vi "Initialize System (Single Bus Multiple Lines).vi"(0 "bus configuration":T1={"nominal voltage [V]"=230.0, "nominal frequency"=enum."50 Hz", "samples per cycle"=192, "type of reference voltage"=enum."Constant", "symmetrical components calculation"=1, "voltage channels"=[], "current channels"=[]} {"current channels"."physical channels"."channel phase" items=["Phase A (L1)", "Phase B (L2)", "Phase C (L3)", "Phase N (Neutral)"]; "voltage channels"."physical channels"."channel phase" items=["Phase A (L1)", "Phase B (L2)", "Phase C (L3)", "Phase N (Neutral)"]; "symmetrical components calculation" items=["Phase to Phase", "Phase to Neutral"]; "samples per cycle" min=128 max=512}, 11 "error in (no error)":errorcluster) -> (4 "nominal sample rate [Hz]":u16, 10 "system info out":refnum<class "EP System Info.lvclass">, 15 "error out":errorcluster)   [LabVIEW 2014, in "NI_EP_Power Quality.lvlib"]
doc: "Sets the basic configuration of the electrical power system based on different line and bus configurations. You must manually select the polymorphic instance you want to use."
uses:
  <vilib>/addons/Electrical Power/PQ/NI_EP_Power Quality.lvlib
  <vilib>/addons/Electrical Power/PQ/Common/Classes/System Info/EP System Info.lvclass
  <vilib>/addons/Electrical Power/PQ/Common/Controls/ep_Bus Config.ctl
  <vilib>/addons/Electrical Power/PQ/Common/Controls/ep_Symmetrical Component Calculation.ctl
  <vilib>/addons/Electrical Power/PQ/Common/Controls/ep_Channels Config.ctl
  <vilib>/addons/Electrical Power/PQ/Common/Controls/ep_Channel Phase.ctl
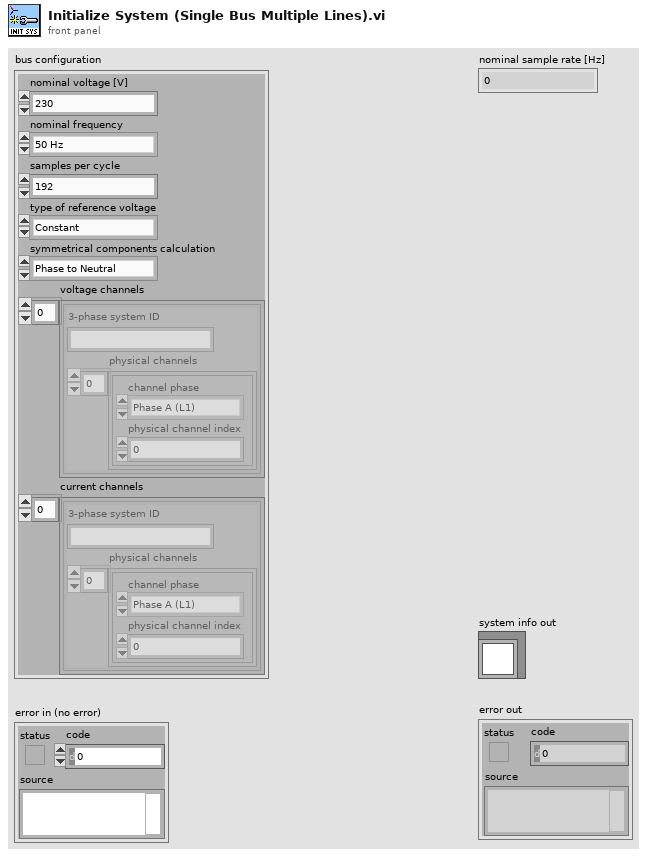
[diagram p1: front panel]
types:
  T1 = typedef "NI_EP_Power Quality.lvlib/ep_Bus Config.ctl" = cluster{"nominal voltage [V]":dbl, "nominal frequency":enum16{"50 Hz", "60 Hz"}, "samples per cycle":u16, "type of reference voltage":enum16{"Constant", "Sliding"}, "symmetrical components calculation":T2, "voltage channels":T3[], "current channels":T3[]}
  T2 = typedef "NI_EP_Power Quality.lvlib/ep_Symmetrical Component Calculation.ctl" = u16
  T3 = typedef "NI_EP_Power Quality.lvlib/ep_Channels Config.ctl" = cluster{"3-phase system ID":string, "physical channels":cluster{"channel phase":T4, "physical channel index":u16}[]}
  T4 = typedef "NI_EP_Power Quality.lvlib/ep_Channel Phase.ctl" = u16
  T5 = typedef "NI_EP_Power Quality.lvlib/ep_Channel Ranges.ctl" = cluster{"3-phase system ID":string, "ranges":dbl[]}
  T6 = typedef "NI_EP_Power Quality.lvlib/ep_Channel Sensitivity.ctl" = cluster{"3-phase system ID":string, "sensitivity":dbl[]}
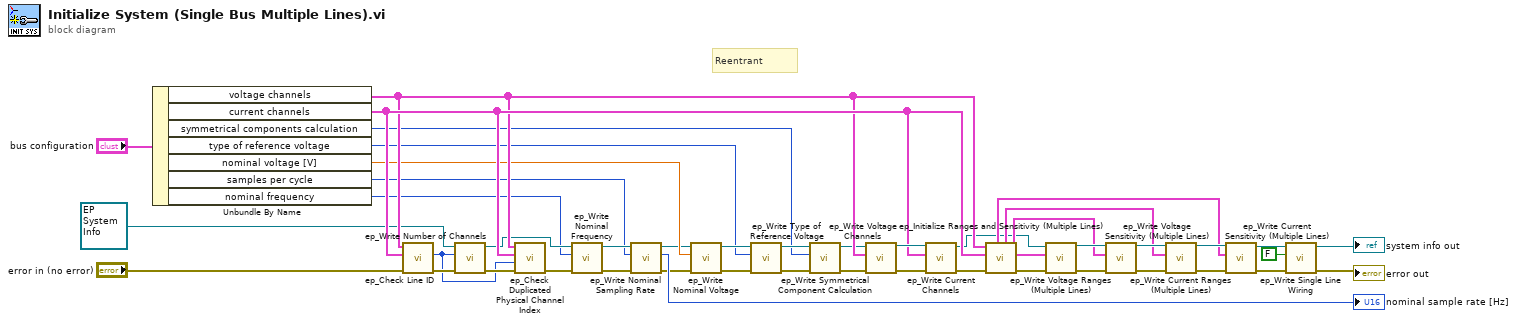
[diagram p0: block diagram]
diagram:
  # "Reentrant"
  n1 = Unbundle By Name("bus configuration") -> ("voltage channels"=w34:T3[], "current channels"=w35:T3[], "symmetrical components calculation"=w10:T2, "type of reference voltage"=w21:enum16{"Constant", "Sliding"}, "nominal voltage [V]"=w22:dbl, "samples per cycle"=w2:u16, "nominal frequency"=w7:enum16{"50 Hz", "60 Hz"})
  n2 = call <vilib>:"ep_Check Line ID.vi"("error in (no error)"="error in (no error)", "current channels"=w35, "voltage channels"=w34) -> ("error out"=w18:errorcluster, "number of channels"=w15:i32)  [unwired: 7 in]
  n3 = call <vilib>:"ep_Write Number of Channels.vi"("error in (no error)"=w18, "number of channels"=w15, "system info in"=refnum<class "EP System Info.lvclass"> refnum ("EP System Info.lvclass")) -> ("error out"=w17:errorcluster, "system info out"=w8:refnum<class "EP System Info.lvclass">)  [unwired: 7 in]
  n4 = call <vilib>:"ep_Check Duplicated Physical Channel Index.vi"("error in (no error)"=w17, "number of channels"=w15, "current channels"=w35, "voltage channels"=w34) -> ("error out"=w9:errorcluster)  [unwired: 7 in]
  n5 = call <vilib>:"ep_Write Nominal Frequency.vi"("error in (no error)"=w9, "nominal frequency"=w7, "system info in"=w8) -> ("error out"=w6:errorcluster, "system info out"=w4:refnum<class "EP System Info.lvclass">)  [unwired: 7 in]
  n6 = call <vilib>:"ep_Write Nominal Sampling Rate.vi"("error in (no error)"=w6, "samples per cycle"=w2, "system info in"=w4) -> ("error out"=w5:errorcluster, "nominal sampling rate [Hz]"=→"nominal sample rate [Hz]":u16, "system info out"=w3:refnum<class "EP System Info.lvclass">)  [unwired: 6 in]
  n7 = call <vilib>:"ep_Write Nominal Voltage.vi"("error in (no error)"=w5, "nominal voltage [V]"=w22, "system info in"=w3) -> ("error out"=w45:errorcluster, "system info out"=w46:refnum<class "EP System Info.lvclass">)  [unwired: 7 in]
  n8 = call <vilib>:"ep_Write Type of Reference Voltage.vi"("error in (no error)"=w45, "type of reference voltage"=w21, "system info in"=w46) -> ("error out"=w13:errorcluster, "system info out"=w14:refnum<class "EP System Info.lvclass">)  [unwired: 7 in]
  n9 = call <vilib>:"ep_Write Symmetrical Component Calculation.vi"("error in (no error)"=w13, "symmetrical component calculation"=w10, "system info in"=w14) -> ("error out"=w12:errorcluster, "system info out"=w11:refnum<class "EP System Info.lvclass">)  [unwired: 7 in]
  n10 = call <vilib>:"ep_Write Voltage Channels.vi"("error in (no error)"=w12, "voltage channels"=w34, "system info in"=w11) -> ("error out"=w36:errorcluster, "system info out"=w37:refnum<class "EP System Info.lvclass">)  [unwired: 7 in]
  n11 = call <vilib>:"ep_Write Current Channels.vi"("error in (no error)"=w36, "current channels"=w35, "system info in"=w37) -> ("error out"=w29:errorcluster, "system info out"=w20:refnum<class "EP System Info.lvclass">)  [unwired: 7 in]
  n12 = call <vilib>:"ep_Initialize Ranges and Sensitivity (Multiple Lines).vi"("error in (no error)"=w29, "current channels"=w35, "voltage channels"=w34) -> ("error out"=w19:errorcluster, "voltage ranges"=w30:T5[], "voltage sensitivity"=w31:T6[], "current ranges"=w32:T5[], "current sensitivity"=w33:T6[])  [unwired: 4 in]
  n13 = call <vilib>:"ep_Write Voltage Ranges (Multiple Lines).vi"("error in (no error)"=w19, "voltage ranges (multiline)"=w30, "system info in"=w20) -> ("error out"=w44:errorcluster, "system info out"=w41:refnum<class "EP System Info.lvclass">)  [unwired: 7 in]
  n14 = call <vilib>:"ep_Write Voltage Sensitivity (Multiple Lines).vi"("error in (no error)"=w44, "voltage sensitivity (multiline)"=w31, "system info in"=w41) -> ("error out"=w43:errorcluster, "system info out"=w40:refnum<class "EP System Info.lvclass">)  [unwired: 7 in]
  n15 = call <vilib>:"ep_Write Current Ranges (Multiple Lines).vi"("error in (no error)"=w43, "current ranges (multiline)"=w32, "system info in"=w40) -> ("error out"=w42:errorcluster, "system info out"=w39:refnum<class "EP System Info.lvclass">)  [unwired: 7 in]
  n16 = call <vilib>:"ep_Write Current Sensitivity (Multiple Lines).vi"("error in (no error)"=w42, "current sensitivity (multiline)"=w33, "system info in"=w39) -> ("error out"=w26:errorcluster, "system info out"=w27:refnum<class "EP System Info.lvclass">)  [unwired: 7 in]
  n17 = call <vilib>:"ep_Write Single Line Wiring.vi"("error in (no error)"=w26, "single line wiring? (F)"=FALSE, "system info in"=w27) -> ("error out"=→"error out":errorcluster, "system info out"=→"system info out":refnum<class "EP System Info.lvclass">)  [unwired: 7 in]
